vi "Matrix Transpose and Print Result.vi"() -> ()   [LabVIEW 2014, in "Arduino MatrixMath.lvlib"]
uses:
  Arduino MatrixMath.lvlib
  <vilib>/LabVIEW Universal Transcriptor/LabVIEW for Arduino SoftwareSerial Library/Arduino SoftwareSerial Wrapper.lvlib
panel:
  in  "A":sgl[](array[numeric])=[1.0, 0.0, 0.0, 1.0, 1.0, 0.0, 0.0, 0.0, 0.0]
  out "Error Out":errorcluster
  in  "Error In":errorcluster
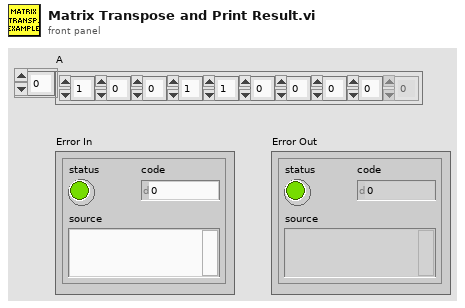
[diagram p1: front panel]
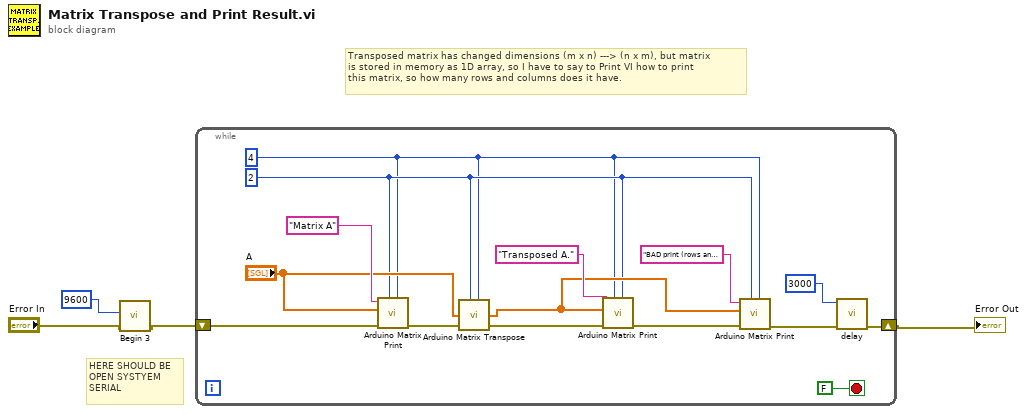
[diagram p0: block diagram]
diagram:
  # "HERE SHOULD BE\nOPEN SYSTYEM\nSERIAL"
  # "Transposed matrix has changed dimensions (m x n) ---> (n x m), but matrix\nis stored in memory as 1D array, so I have to say to Print VI how to print\nthis matrix, so how many rows and columns does it have."
  n1 = call <vilib>:"Begin 3.vi"("Error In"="Error In", "Baudrate"=u16 9600 ("Speed")) -> ("Error Out"=w4:errorcluster)  [unwired: 8 in]
  n2 = while {
    shift-right: [w7] -> w1
    shift-left: w4 -> [w18]
    stop <- FALSE stop-if-true
    w8 = u8 4 ("cols num.")
    w9 = u8 2 ("rows num.")
    n3 = call "Arduino Matrix Print.vi"("cols num."=w8, "rows num."=w9, "Error In"=w18, "A"="A", "Label"="Matrix A") -> ("Error Out"=w15:errorcluster)  [unwired: 6 in]
    n4 = call "Arduino Matrix Transpose.vi"("rows num."=w9, "A"="A", "Error In"=w15, "cols num."=w8) -> ("transposed A"=w10:sgl[], "Error Out"=w14:errorcluster)  [unwired: 4 in]
    n5 = call "Arduino Matrix Print.vi"("cols num."=w9, "rows num."=w8, "Error In"=w14, "A"=w10, "Label"="Transposed A.") -> ("Error Out"=w12:errorcluster)  [unwired: 6 in]
    n6 = call "Arduino Matrix Print.vi"("cols num."=w8, "rows num."=w9, "Error In"=w12, "A"=w10, "Label"="BAD print (rows and cols siwtched)") -> ("Error Out"=w6:errorcluster)  [unwired: 6 in]
    n7 = call <vilib>:"delay.vi"("Error In"=w6, "time (ms)"=3000 ("delay")) -> ("Error Out"=w7:errorcluster)  [unwired: 9 in]
  }
  "Error Out" <- w1
